vi "Unpack and Repack Package.vi"() -> ()   [LabVIEW 2015]
panel:
  out "error out":errorcluster
  in  "error in (no error)":errorcluster
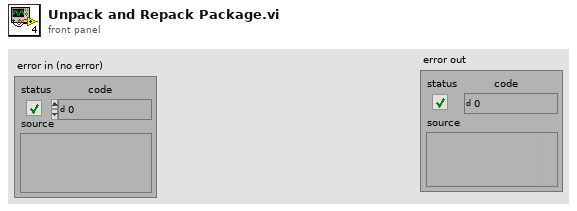
[diagram p1: front panel]
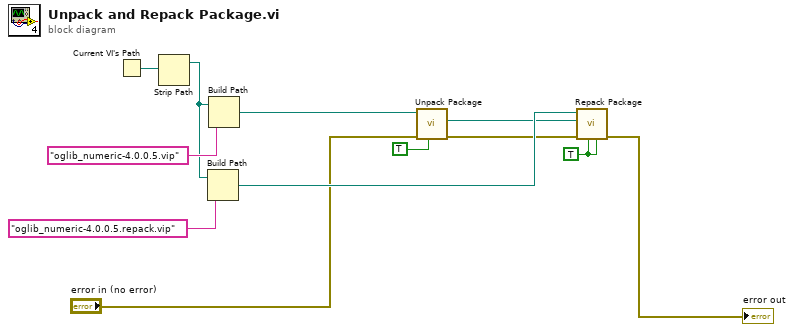
[diagram p0: block diagram]
diagram:
  w1 = TRUE ("Delete Directory to repack (if success)?")
  n1 = Current VI's Path() -> (path=w12:path)
  n2 = Strip Path(path=w12) -> (stripped path=w7:path)  [unwired: 1 out]
  n3 = Build Path(base path=w7, name or relative path="oglib_numeric-4.0.0.5.repack.vip") -> (appended path=w6:path)
  n4 = Build Path(base path=w7, name or relative path="oglib_numeric-4.0.0.5.vip") -> (appended path=w10:path)
  n5 = call "Unpack Package.vi"("Overwrite Target Directory (if exists)?"=TRUE, "error in (no error)"="error in (no error)", "Package File"=w10) -> ("error out"=w4:errorcluster, "Unpacked Package Directory"=w5:path)  [unwired: 5 in, 2 out]
  n6 = call "Repack Package.vi"("Delete Directory to repack (if success)?"=w1, "Overwrite Target Package File (if exists)?"=w1, "error in (no error)"=w4, "Directory to repack"=w5, "Package File"=w6) -> ("error out"=→"error out":errorcluster)  [unwired: 5 in, 1 out]
